vi "Local_xy_graph.vi"(9 "x_lat_path":dbl[](array[numeric]), 10 "y_long_path":dbl[](array[numeric]), 11 "XYGraph in":refnum<vi>) -> ()   [LabVIEW 2015]
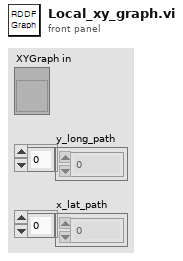
[diagram p1: front panel]
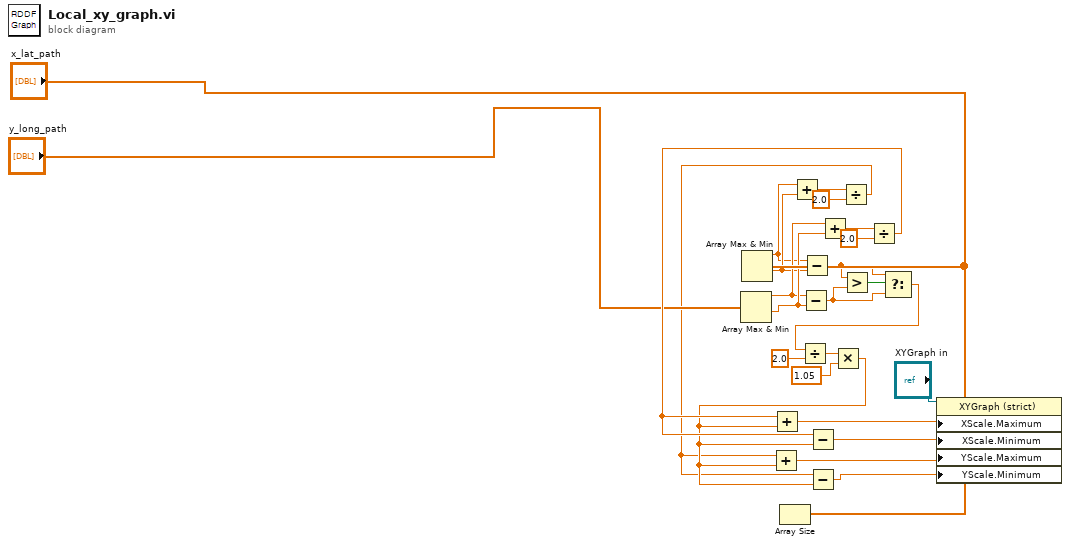
[diagram p0: block diagram]
diagram:
  n1 = Array Max & Min(array="y_long_path") -> (max value=w13:dbl, min value=w14:dbl)  [unwired: 2 out]
  n2 = Array Max & Min(array="x_lat_path") -> (max value=w7:dbl, min value=w8:dbl)  [unwired: 2 out]
  n3 = Array Size(array="x_lat_path") -> ()  [unwired: 1 out]
  n4 = Add(x=w7, y=w8) -> (x+y=w10:dbl)
  n5 = Subtract(x=w13, y=w14) -> (x-y=w4:dbl)
  n6 = Subtract(x=w7, y=w8) -> (x-y=w3:dbl)
  n7 = Add(x=w13, y=w14) -> (x+y=w11:dbl)
  n8 = Divide(x=w10, y=2.0) -> (x/y=w17:dbl)
  n9 = Greater?(x=w3, y=w4) -> (0:w2:bool)
  n10 = Divide(x=w11, y=2.0) -> (x/y=w25:dbl)
  n11 = Select(t=w3, s=w2, f=w4) -> (s? t:f=w6:dbl)
  n12 = Divide(x=w6, y=2.0) -> (x/y=w15:dbl)
  n13 = Multiply(x=w15, y=1.05) -> (x*y=w18:dbl)
  n14 = Add(x=w17, y=w18) -> (x+y=w20:dbl)
  n15 = Add(x=w25, y=w18) -> (x+y=w22:dbl)
  n16 = Subtract(x=w25, y=w18) -> (x-y=w21:dbl)
  n17 = Subtract(x=w17, y=w18) -> (x-y=w19:dbl)
  n18 = property on="Property Node" class="XYGraph (strict)"(reference="XYGraph in", "XScale.Maximum"=w22, "XScale.Minimum"=w21, "YScale.Maximum"=w20, "YScale.Minimum"=w19) -> ()  [unwired: 1 in, 2 out]
